vi "Add Sniffer Callback.vi"(7 "Owner":refnum<class>, 8 "error in (no error)":errorcluster, 10 "Callback":refnum<vi>, 11 "Endpoint in":refnum<class "Endpoint.lvclass">) -> (0 "error out":errorcluster, 3 "Endpoint out":refnum<class "Endpoint.lvclass">)   [LabVIEW 2020, in "Stream.lvlib" / "Endpoint.lvclass"]
uses:
  Endpoint.lvclass
  State Callback.ctl
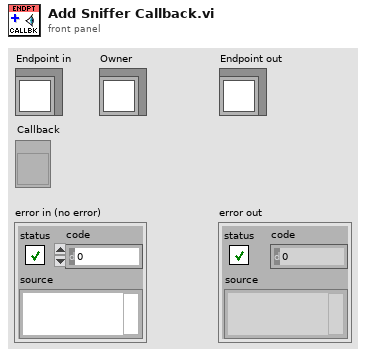
[diagram p1: front panel]
types:
  T1 = typedef "Stream.lvlib/Endpoint.lvclass/State Callback.ctl" = cluster{"Owner":refnum<class>, "VI":refnum<vi>, "Context":variant}
  T2 = typedef "Stream.lvlib/Endpoint.lvclass/Ref Data.ctl" = cluster{"URI":refnum<class "URI.lvclass">, "State Callbacks":T1[], "Sniffer Callbacks":T1[]}
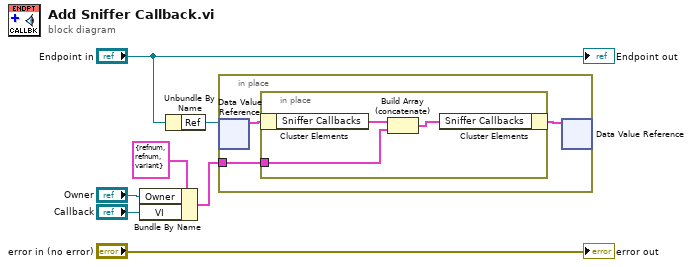
[diagram p0: block diagram]
diagram:
  n1 = Bundle By Name(cluster=T1 {"Owner"=refnum, "VI"=refnum, "Context"=variant} ("State Callback"), "Owner"="Owner", "VI"="Callback") -> (w3:T1)
  n2 = Unbundle By Name("Endpoint in") -> ("Ref"=w6:refnum<data-value>)
  n3 = in-place {
    in-place-border: w3 -> [w8]
    n4 = in-place-dvr #1(w6) -> (w10:T2)  [unwired: 1 out]
    n5 = in-place {
      in-place-border: w8 -> [w12]
      n6 = in-place-cluster #2(w10) -> ("Sniffer Callbacks"=w13:T1[])
      n7 = Build Array (concatenate)(w13, w12) -> (w11:T1[])
      n8 = in-place-cluster #2("Sniffer Callbacks"=w11) -> (w9:T2)
    }
    n9 = in-place-dvr #1(w9) -> ()  [unwired: 2 out]
  }
  "error out" <- "error in (no error)"
  "Endpoint out" <- "Endpoint in"
